vi "DriveSetRobotPosition.vi"(2 "Parameter String":string, 3 "Reinit":bool) -> (0 "Error Out":errorcluster, 1 "Increment":bool)   [LabVIEW 2020]
doc: "This VI sets the robot position. This can be used to zero out accumulated position error based on a fiducial.\n\nParameters:\n1. X location --> (in) [0,648]\n2. Y location --> (in) [0,324]"
uses:
  SafeParser_Float.vi
  GlobalPoseAndTargeting.vi
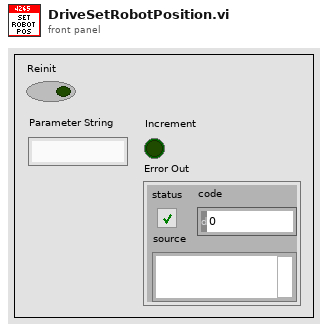
[diagram p1: front panel]
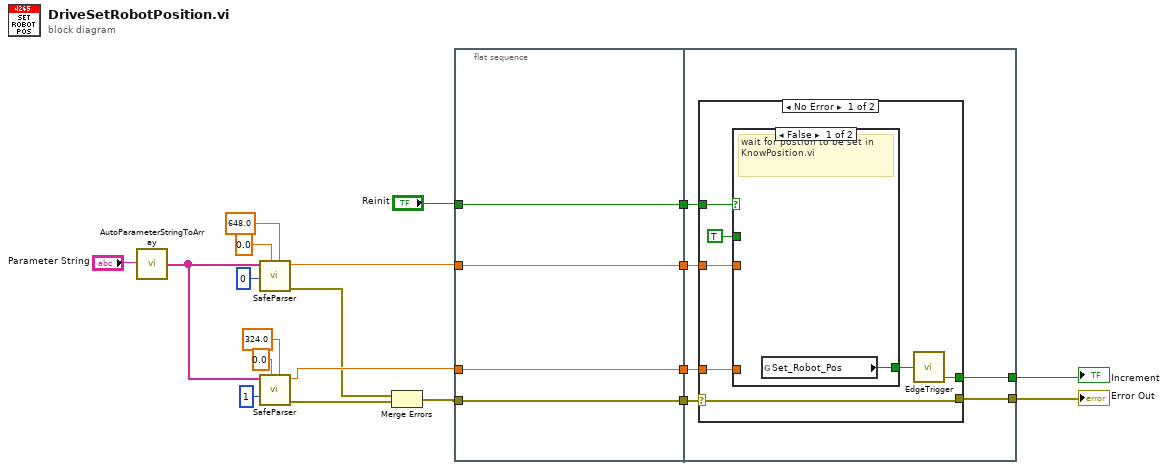
[diagram p0: block diagram]
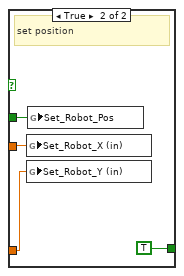
[diagram p2: hidden frame]
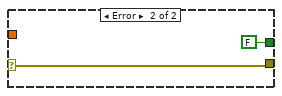
[diagram p3: hidden frame]
diagram:
  n1 = call "AutoParameterStringToArray.vi"("Parameter String"="Parameter String") -> ("Parsed Parameters"=w13:string[])
  n2 = call-poly "SafeParser.vi"("Maximum"=648.0, "Minimum"=0.0, "Array Index"=0 ("Parameter Index"), "String Array"=w13) -> ("Error Out"=w7:errorcluster, "Typecast  Value"=w9:dbl)  [unwired: 6 in]
  n3 = call-poly "SafeParser.vi"("Maximum"=324.0, "Minimum"=0.0, "Array Index"=1 ("Parameter Index"), "String Array"=w13) -> ("Error Out"=w10:errorcluster, "Typecast  Value"=w8:dbl)  [unwired: 6 in]
  n4 = Merge Errors(w7, w10) -> (w11:errorcluster)
  n5 = flat-sequence {
    tunnel: w8 -> [w21]
    tunnel: w9 -> [w22]
    tunnel: w11 -> [w23]
    tunnel: "Reinit" -> [w24]
    tunnel: [w24] -> w4
    tunnel: [w23] -> w3
    tunnel: [w22] -> w2
    tunnel: [w21] -> w1
    tunnel: [w29] -> w19
    tunnel: [w28] -> w18
    tunnel: w4 -> [w30]
    tunnel: w3 -> [w27]
    tunnel: w2 -> [w26]
    tunnel: w1 -> [w25]
    frame #0 {
    }
    frame #1 {
      n6 = case shown="No Error" w27 {
        selector: w27 -> [w32 w44]
        tunnel: w30 -> [w37 _]
        tunnel: w26 -> [w36 _]
        tunnel: [w33 FALSE ("Falling Edge Trigger")] -> w29
        tunnel: [w32 w44] -> w28
        tunnel: w25 -> [w31 _]
        frame No Error {
          n7 = case shown="False" w37 {
            tunnel: w36 -> [_ w42]
            tunnel: [w38 TRUE ("Falling Edge Trigger")] -> w34
            tunnel: TRUE -> [_ w40]
            tunnel: w31 -> [_ w39]
            frame False {
              # "wait for postion to be set in KnowPosition.vi"
              n8 = global read "GlobalPoseAndTargeting.vi" "Set_Robot_Pos"() -> (w38:bool)
            }
            frame True {
              # "set position"
              n9 = global write "GlobalPoseAndTargeting.vi" "Set_Robot_X (in)"(w42) -> ()
              n10 = global write "GlobalPoseAndTargeting.vi" "Set_Robot_Y (in)"(w39) -> ()
              n11 = global write "GlobalPoseAndTargeting.vi" "Set_Robot_Pos"(w40) -> ()
            }
          }
          n12 = call "EdgeTrigger.vi"("Input Signal"=w34) -> ("Falling Edge Trigger"=w33:bool)  [unwired: 2 out]
        }
        frame Error {
        }
      }
    }
  }
  "Increment" <- w19
  "Error Out" <- w18
